vi "setZoomTool.vi"(9 "Zoom Y":bool, 10 "Zoom  X":bool, 11 "reference":refnum<vi>) -> ()   [LabVIEW 2013]
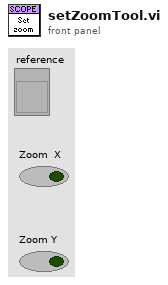
[diagram p1: front panel]
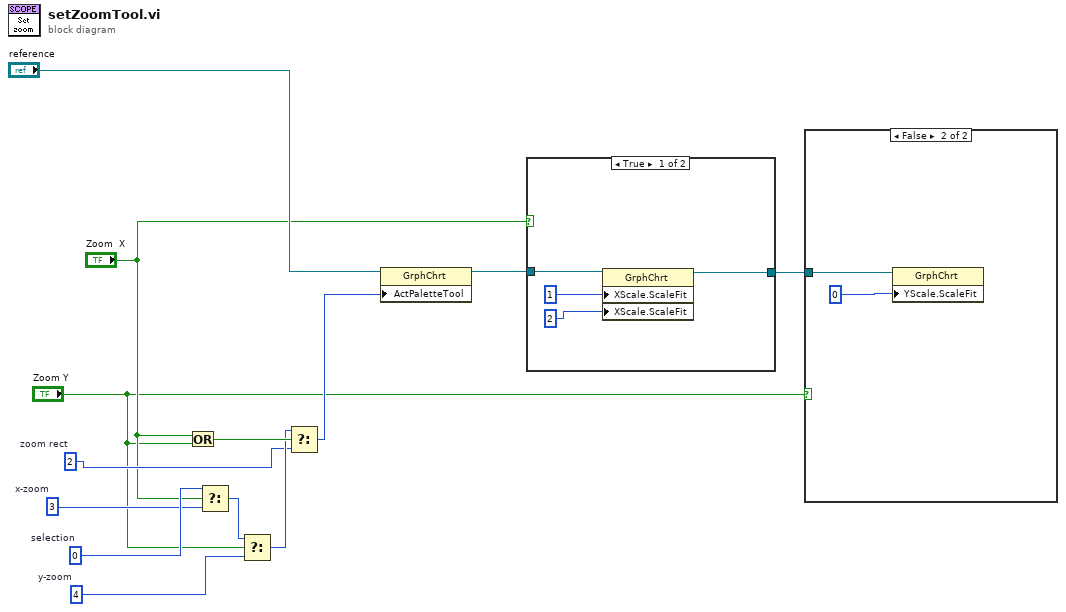
[diagram p0: block diagram]
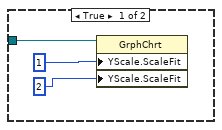
[diagram p2: hidden frame]
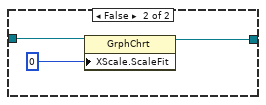
[diagram p3: hidden frame]
diagram:
  w8 = 2  # zoom rect
  w5 = 4  # y-zoom
  w6 = 3  # x-zoom
  w12 = 0  # selection
  n1 = Or(x="Zoom  X", y="Zoom Y") -> (x .or. y?=w11:bool)
  n2 = Select(t=w12, s="Zoom  X", f=w6) -> (s? t:f=w10:i32)
  n3 = Select(t=w10, s="Zoom Y", f=w5) -> (s? t:f=w9:i32)
  n4 = Select(t=w9, s=w11, f=w8) -> (s? t:f=w7:i32)
  n5 = property on="Property Node" class="GrphChrt"(reference="reference", "ActPaletteTool"=w7) -> (reference out=w3:refnum<vi>)  [unwired: 1 in, 1 out]
  n6 = case shown="True" "Zoom  X" {
    tunnel: w3 -> [w17 w20]
    tunnel: [w14 w18] -> w1
    frame True {
      n7 = property on="Property Node" class="GrphChrt"(reference=w17, "XScale.ScaleFit"=u8 1 ("X Scale.Scale Fit"), "XScale.ScaleFit"=u8 2 ("X Scale.Scale Fit")) -> (reference out=w14:refnum<vi>)  [unwired: 1 in, 1 out]
    }
    frame False {
      n8 = property on="Property Node" class="GrphChrt"(reference=w20, "XScale.ScaleFit"=u8 0 ("X Scale.Scale Fit")) -> (reference out=w18:refnum<vi>)  [unwired: 1 in, 1 out]
    }
  }
  n9 = case shown="False" "Zoom Y" {
    tunnel: w1 -> [w23 w25]
    frame True {
      n10 = property on="Property Node" class="GrphChrt"(reference=w23, "YScale.ScaleFit"=u8 1 ("X Scale.Scale Fit"), "YScale.ScaleFit"=u8 2 ("X Scale.Scale Fit")) -> ()  [unwired: 1 in, 2 out]
    }
    frame False {
      n11 = property on="Property Node" class="GrphChrt"(reference=w25, "YScale.ScaleFit"=u8 0 ("X Scale.Scale Fit")) -> ()  [unwired: 1 in, 2 out]
    }
  }
